vi "_Raise Navigation Starting Event.vi"(4 "WebView2.lvlib:WebView2 Control.lvclass":refnum<class "WebView2 Control.lvclass">, 5 "Event Data":cluster{"sender":refnum<k24>, "e":refnum<k24>}, 6 "Control Ref":refnum<k24>, 7 "Event Common Data":T1) -> ()   [LabVIEW 2020, in "WebView2.lvlib" / "WebView2 Control.lvclass"]
uses:
  WebView2 Control.lvclass
  C:/Users/Simon/Documents/GitHub/LV-WebView2/Source/Libs/Microsoft.Web.WebView2.Core.dll
  Libs/Microsoft.Web.WebView2.Core.dll
  Navigation Start Event Data.ctl
  WebView2 Control.lvclass/WebView2 Control.ctl
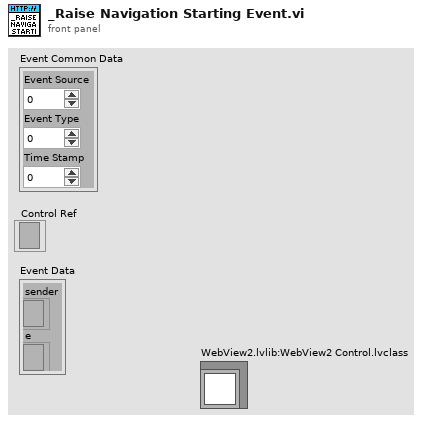
[diagram p1: front panel]
types:
  T1 = cluster{"Event Source":i32, "Event Type":u32, "Time Stamp":u32}
  T2 = typedef "WebView2.lvlib/WebView2 Control.lvclass/Navigation Start Event Data.ctl" = cluster{"AdditionalAllowedFrameAncestors":string, "Cancel":bool, "IsRedirected":bool, "IsUserInitiated":bool, "NavigationId":u64, "NavigationKind":i32, "Uri":string, "Headers":cluster{"Key":string, "Value":string}[]}
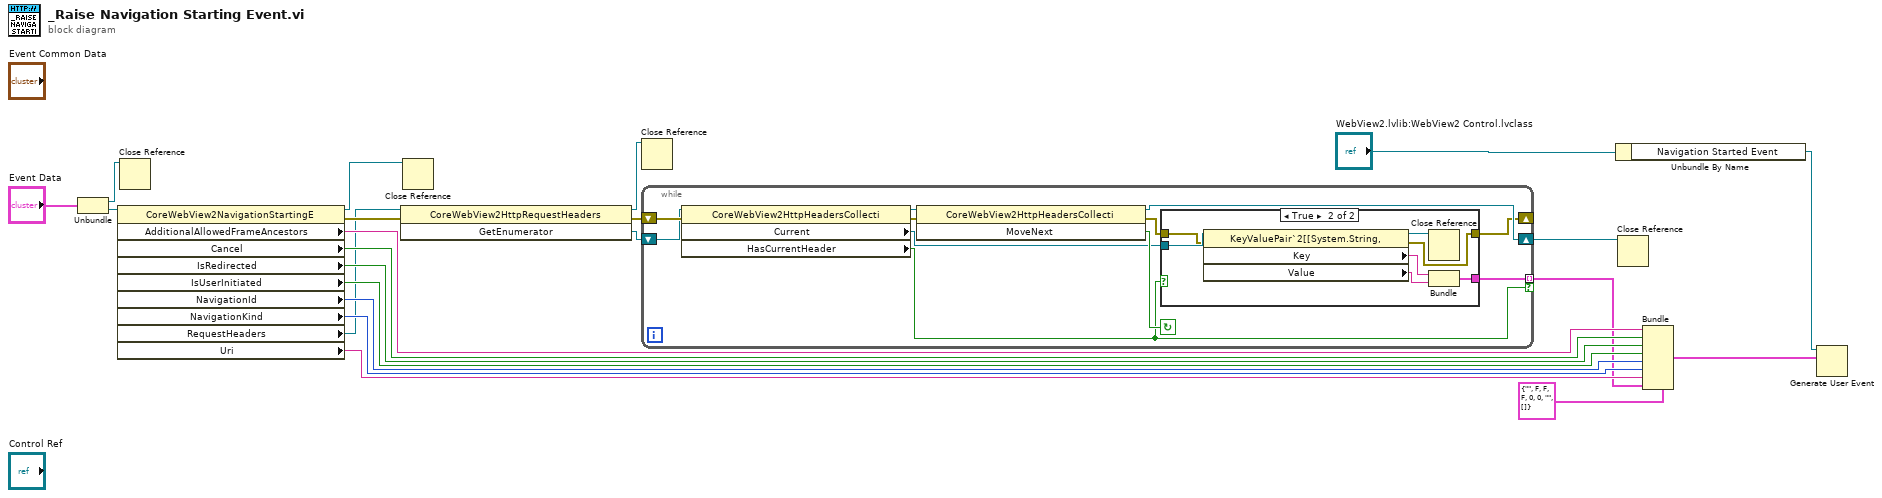
[diagram p0: block diagram]
diagram:
  n1 = Unbundle("Event Data") -> ("sender"=w10:refnum<k24>, "e"=w20:refnum<k24>)
  n2 = property class="CoreWebView2NavigationStartingE"(reference=w20) -> (reference out=w9:refnum<k24>, error out=w3:errorcluster, "AdditionalAllowedFrameAncestors"=w18:string, "Cancel"=w17:bool, "IsRedirected"=w16:bool, "IsUserInitiated"=w15:bool, "NavigationId"=w14:u64, "NavigationKind"=w13:i32, "RequestHeaders"=w1:refnum<k24>, "Uri"=w5:string)  [unwired: 1 in]
  n3 = Close Reference(reference=w10) -> ()  [unwired: 1 in, 1 out]
  n4 = invoke class="CoreWebView2HttpRequestHeaders" method="GetEnumerator"(reference=w1, error in=w3) -> (reference out=w2:refnum<k24>, error out=w7:errorcluster, "GetEnumerator"=w8:refnum<k24>)  [unwired: 1 in]
  n5 = Close Reference(reference=w9) -> ()  [unwired: 1 in, 1 out]
  n6 = Close Reference(reference=w2) -> ()  [unwired: 1 in, 1 out]
  n7 = while {
    shift-right: [w26] -> w6
    shift-left: w8 -> [w30]
    shift-right: [w24] -> _
    shift-left: w7 -> [w32]
    tunnel: [w27] -> w4 mode=indexing if=w23
    stop <- w33 continue-if-true
    n8 = property class="CoreWebView2HttpHeadersCollecti"(reference=w30, error in=w32) -> (reference out=w29:refnum<k24>, error out=w31:errorcluster, "Current"=w28:refnum<k24>, "HasCurrentHeader"=w23:bool)
    n9 = invoke class="CoreWebView2HttpHeadersCollecti" method="MoveNext"(reference=w29, error in=w31) -> (reference out=w26:refnum<k24>, error out=w25:errorcluster, "MoveNext"=w33:bool)  [unwired: 1 in]
    n10 = case shown="True" w23 {
      tunnel: w28 -> [_ w41]
      tunnel: [_ w38] -> w27
      tunnel: w25 -> [w34 w36]
      tunnel: [w34 w35] -> w24
      frame False {
      }
      frame True {
        n11 = property class="KeyValuePair`2[[System.String, "(reference=w41, error in=w36) -> (reference out=w37:refnum<k24>, error out=w35:errorcluster, "Key"=w40:string, "Value"=w39:string)
        n12 = Close Reference(reference=w37) -> ()  [unwired: 1 in, 1 out]
        n13 = Bundle("Key"=w40, "Value"=w39) -> (w38:cluster{"Key":string, "Value":string})  [unwired: 1 in]
      }
    }
  }
  n14 = Unbundle By Name("WebView2.lvlib:WebView2 Control.lvclass") -> ("Navigation Started Event"=w22:refnum<user-event>)
  n15 = Close Reference(reference=w6) -> ()  [unwired: 1 in, 1 out]
  n16 = Bundle(cluster=T2 {"AdditionalAllowedFrameAncestors"="", "Cancel"=FALSE, "IsRedirected"=FALSE, "IsUserInitiated"=FALSE, "NavigationId"=0, "NavigationKind"=0, "Uri"="", "Headers"=[]} ("Nav Started Event"), "AdditionalAllowedFrameAncestors"=w18, "Cancel"=w17, "IsRedirected"=w16, "IsUserInitiated"=w15, "NavigationId"=w14, "NavigationKind"=w13, "Uri"=w5, "Headers"=w4) -> (w11:T2)
  n17 = Generate User Event(user event=w22, event data cluster=w11) -> ()  [unwired: 2 in, 2 out]
